vi "clusters 12 - Copy.vi"() -> ()   [LabVIEW 2025]
panel:
  out "age 2":dbl
  in  "Cluster":T1
  out "age":dbl
  out "second name":string
  out "first name":string
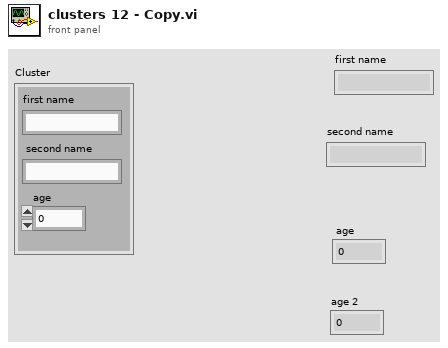
[diagram p1: front panel]
types:
  T1 = cluster{"first name":string, " second name":string, "age":dbl}
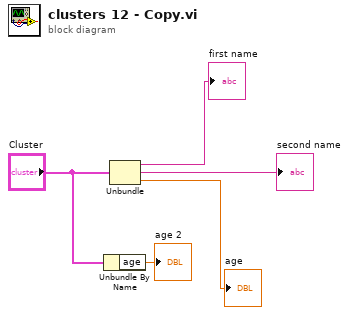
[diagram p0: block diagram]
diagram:
  n1 = Unbundle By Name("Cluster") -> ("age"=→"age 2":dbl)
  n2 = Unbundle("Cluster") -> ("first name"=→"first name":string, "second name"=→"second name":string, "age"=→"age":dbl)
